vi "Get Node Count.vi"(8 "error in":errorcluster, 11 "File Info in":T1) -> (0 "error out":errorcluster, 3 "File Info out":T1)   [LabVIEW 2020, in "Peer Review.lvclass"]
uses:
  Peer Review.lvclass
  TypeDefs/File Info.ctl
  TypeDefs/File State.ctl
  TypeDefs/VI Type.ctl
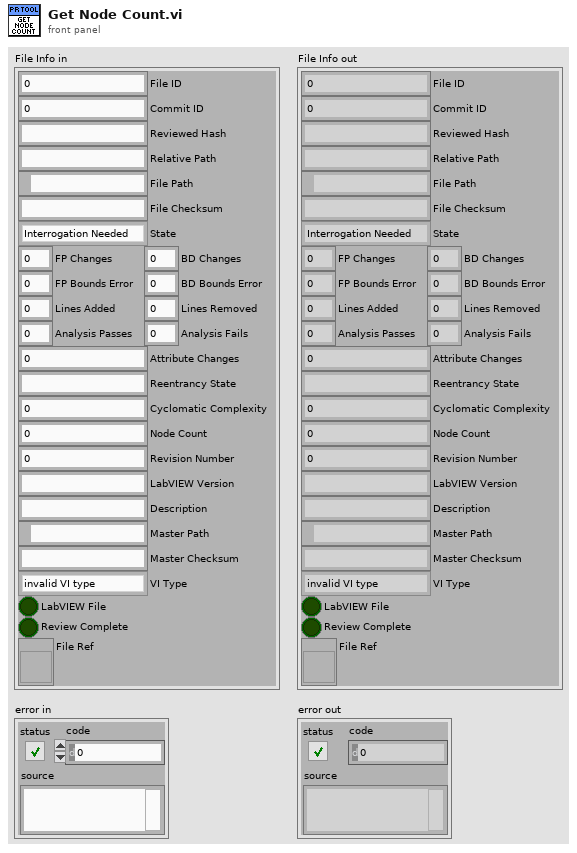
[diagram p1: front panel]
types:
  T1 = typedef "Peer Review.lvclass/File Info.ctl" = cluster{"File ID":i32, "Commit ID":i32, "Reviewed Hash":string, "Relative Path":string, "File Path":path, "File Checksum":string, "State":T2, "FP Changes":i32, "BD Changes":i32, "FP Bounds Error":dbl, "BD Bounds Error":dbl, "Lines Added":i32, "Lines Removed":i32, "Analysis Passes":i32, "Analysis Fails":i32, "Attribute Changes":i32, "Reentrancy State":string, "Cyclomatic Complexity":i32, "Node Count":i32, "Revision Number":u32, "LabVIEW Version":string, "Description":string, "Master Path":path, "Master Checksum":string, "VI Type":T3, "LabVIEW File":bool, "Review Complete":bool, "File Ref":refnum<vi>}
  T2 = typedef "Peer Review.lvclass/File State.ctl" = enum16{"Interrogation Needed", "Modified", "Deleted", "Added", "Matches Previous", "No Changes", "Moved"}
  T3 = typedef "Peer Review.lvclass/VI Type.ctl" = enum32{"invalid VI type", "Standard VI", "Control VI", "Global VI", "Polymorphic VI", "Configuration VI", "SubSystem", "Facade VI", "Method VI", "Statechart Diagram VI"}
  T4 = cluster{"# nodes":u32, "# signals":u32, "# structures":u32, "# diagrams":u32, "diag depth":u32, "# controls":u32, "# indicators":u32, "# inputs":u32, "# outputs":u32, "# global reads":u32, "# global writes":u32, "# local reads":u32, "# local writes":u32, "# attr reads":u32, "# attr writes":u32, "# cins":u32, "# dlls":u32, "diagram width":u32, "diagram height":u32}
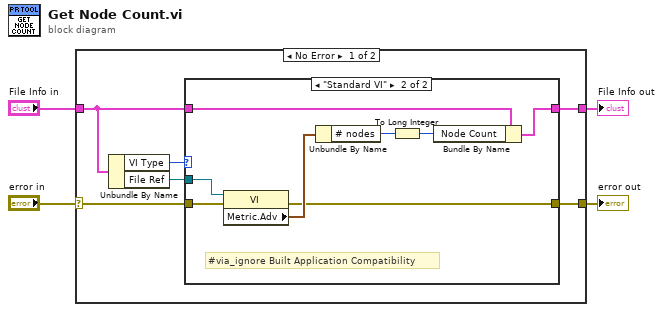
[diagram p0: block diagram]
diagram:
  n1 = case shown="No Error" "error in" {
    selector: "error in" -> [w8 w22]
    tunnel: [w10 w22] -> w4
    tunnel: "File Info in" -> [w7 w21]
    tunnel: [w6 w21] -> w1
    frame No Error {
      n2 = Unbundle By Name(w7) -> ("VI Type"=w9:T3, "File Ref"=w5:refnum<vi>)
      n3 = case shown="\"Standard VI\"" w9 {
        tunnel: [w12 w15] -> w10
        tunnel: w8 -> [w12 w17]
        tunnel: w7 -> [w11 w20]
        tunnel: [w11 w19] -> w6
        tunnel: w5 -> [_ w14]
        frame Default {
        }
        frame "Standard VI" {
          # "#via_ignore Built Application Compatibility"
          n4 = property on="Property Node" class="VI"(reference=w14, error in=w17) -> (error out=w15:errorcluster, "Metric.Adv"=w18:T4)  [unwired: 1 out]
          n5 = Unbundle By Name(w18) -> ("# nodes"=w16:u32)
          n6 = To Long Integer(number=w16) -> (32bit integer=w13:i32)
          n7 = Bundle By Name(cluster=w20, "Node Count"=w13) -> (w19:T1)
        }
      }
    }
    frame Error {
    }
  }
  "error out" <- w4
  "File Info out" <- w1
